vi "test_TCP_1_ Host__v0,02.vi"() -> ()   [LabVIEW 2014]
panel:
  out "accumRead":string
  out "error out":errorcluster
  out "currentRead":string
  in  "stop":bool
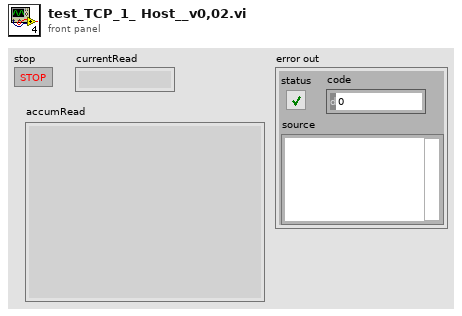
[diagram p1: front panel]
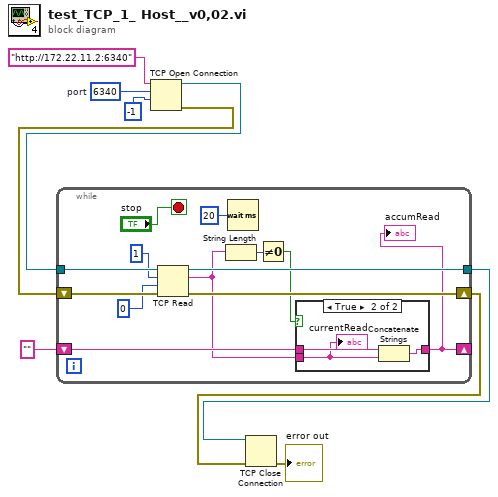
[diagram p0: block diagram]
diagram:
  w5 = u16 6340  # port
  n1 = TCP Open Connection(address="http://172.22.11.2:6340", remote port or service name=w5, timeout ms (60000)=-1) -> (connection ID=w4:refnum<k5>, error out=w3:errorcluster)  [unwired: 2 in]
  n2 = while {
    tunnel: w4 -> [w20]
    shift-right: [w16] -> w8
    shift-left: w3 -> [w19]
    tunnel: [w15] -> w7
    shift-right: [w10] -> _
    shift-left: "" -> [w12]
    stop <- "stop" stop-if-true
    n3 = TCP Read(connection ID=w20, bytes to read=1, error in (no error)=w19, 9:0 ("timeout ms (25000)")) -> (connection ID out=w15:refnum<k5>, data out=w11:string, error out=w16:errorcluster)  [unwired: 1 out]
    n4 = String Length(string=w11) -> (length=w14:i32)
    n5 = Wait (ms)(milliseconds to wait=u32 20) -> ()  [unwired: 1 out]
    n6 = Not Equal To 0?(x=w14) -> (x != 0?=w13:bool)
    n7 = case shown="True" w13 {
      tunnel: w12 -> [w23 w26]
      tunnel: w11 -> [_ w24]
      tunnel: [w23 w25] -> w10
      frame False {
      }
      frame True {
        n8 = Concatenate Strings(w26, w24) -> (w25:string)
        "currentRead" <- w24
      }
    }
    "accumRead" <- w10
  }
  n9 = TCP Close Connection(connection ID=w7, error in (no error)=w8) -> (error out=→"error out":errorcluster)  [unwired: 2 out]
